vi "FSK_Sync.vi"(8 "error in (no error)":errorcluster caption="错误输入（无错误）", 10 "RecvFskDemod":cdb[](array[numeric]), 11 "PathIn":path) -> (0 "error out":errorcluster caption="错误输出", 1 "pos":dbl format="%#_13g", 2 "RecvCorr":dbl[](array[numeric]) format="%#_13g", 3 "PathOut":path)   [LabVIEW 2015]
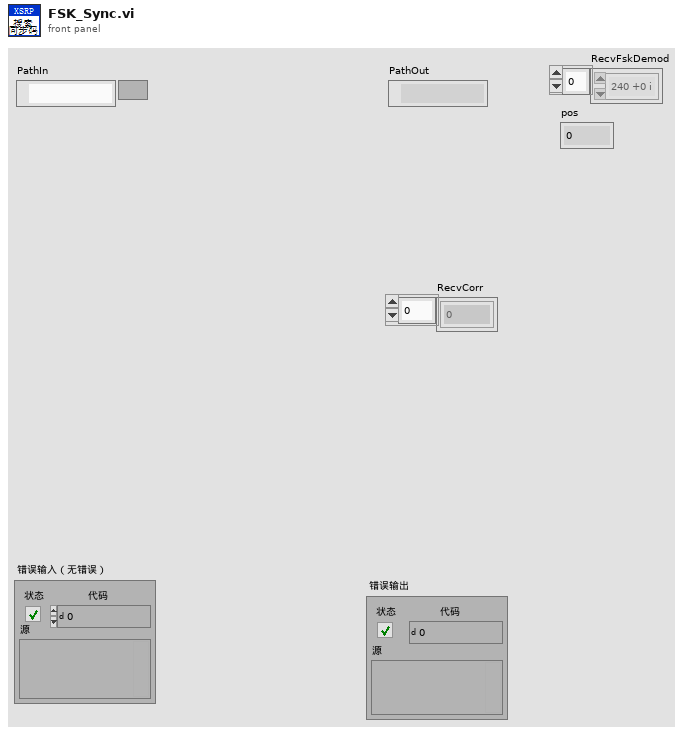
[diagram p1: front panel]
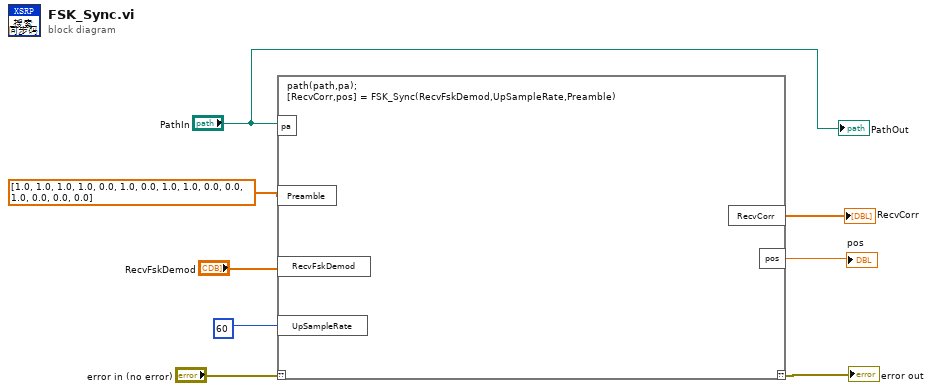
[diagram p0: block diagram]
diagram:
  n1 = script code="path(path,pa);\n[RecvCorr,pos] = FSK_Sync(RecvFskDemod,UpSampleRate,Preamble)"("??"="error in (no error)", "pa"="PathIn", "RecvFskDemod"="RecvFskDemod", "UpSampleRate"=60, "Preamble"=dbl[] [1.0, 1.0, 1.0, 1.0, 0.0, 1.0, 0.0, 1.0, 1.0, 0.0, 0.0, 1.0, 0.0, 0.0, 0.0]) -> ("??"=→"error out":errorcluster, "RecvCorr"=→"RecvCorr":dbl[], "pos"=→"pos":dbl)
  "PathOut" <- "PathIn"
